vi "NCD Update Settings Single.vi"   [LabVIEW 2020]
uses:
  MRC Module.lvlib
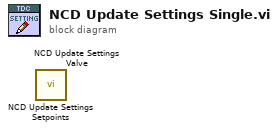
[diagram p0: block diagram]
diagram:
  n1 = call "NCD Update Settings Setpoints.vi"() -> ()  [unwired: 8 in, 4 out]
  n2 = call "NCD Update Settings Valve.vi"() -> ()  [unwired: 9 in, 3 out]
